vi "Manual User Input.vi"() -> (2 "XML":path, 3 "ZIP":path, 4 "Cancelled?":bool=TRUE)   [LabVIEW 2020]
doc: "<p>Select <strong>Tools<span class=\"U+187\">>></span>Synchronize with ni.com Icon Library</strong> from the <a href=\"nihelplauncher://docs/csh?context=lvcore_lvdialog_icon_editor\">Icon Editor</a> dialog box to display the <a href=\"nihelplauncher://docs/csh?context=lvcore_lvdialog_synch_icon_library_db\">Synchronize with Icon Library</a> dialog box. If LabVIEW cannot reach the National Instruments Web server, LabVIEW displays this dialog box.</p>\n\n<p>Use this dialog box to synchronize the <span class=\"Monospace\">LabVIEW Data\\Glyphs</span> directory <a href=\"nihelplauncher://docs/csh?context=lvcore_lvhowto_synchronizing_icon_library\">manually</a> with the most recent glyphs in the <a href=\"https://www.ni.com/r/expnr7\">Icon Library</a> at <span class=\"Monospace\">ni.com</span>.</p>\n\n<p>This dialog box includes the following components:</p>"
panel:
  in  "Loc string":string="LabVIEW cannot reach the National Instruments Web server. You must synchronize with the Icon Library manually.\nClick the Help button for more information about resolving this error."
  in  "Help":bool
  in  "Icon library XML file":path
  in  "Icon library ZIP file":path
  out "Instructions":string
  in  "Cancel":bool
  in  "OK":bool
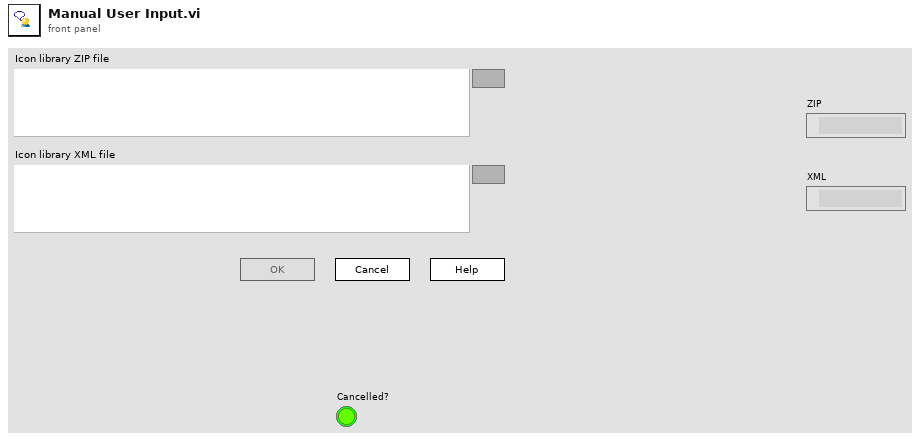
[diagram p1: front panel]
types:
  T1 = enum8{"Enabled", "Disabled", "Disabled and Grayed Out"}
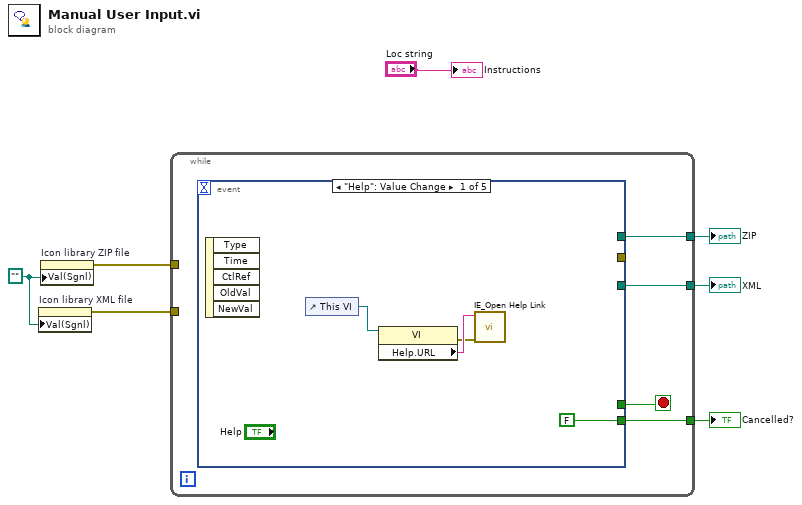
[diagram p0: block diagram]
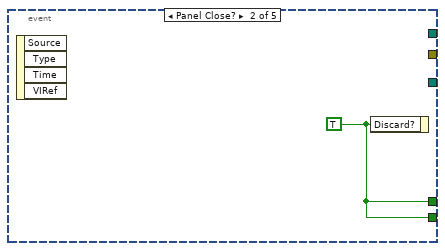
[diagram p2: hidden frame]
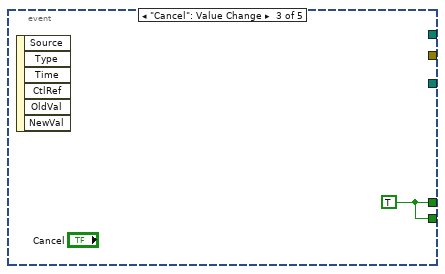
[diagram p3: hidden frame]
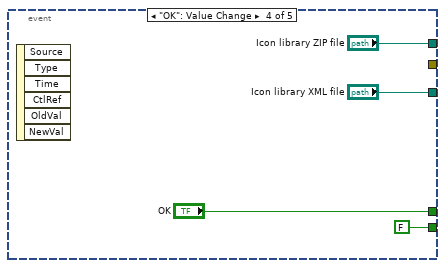
[diagram p4: hidden frame]
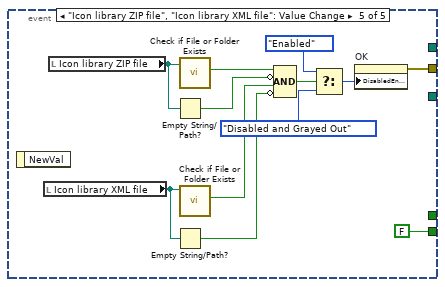
[diagram p5: hidden frame]
diagram:
  w5 = path ""
  n1 = property on="Icon library XML file" class="Path"("Val(Sgnl)"=w5) -> (error out=w2:errorcluster)  [unwired: 2 in, 1 out]
  n2 = property on="Icon library ZIP file" class="Path"("Val(Sgnl)"=w5) -> (error out=w3:errorcluster)  [unwired: 2 in, 1 out]
  n3 = while {
    tunnel: [w8] -> w7
    tunnel: [w11] -> w4
    tunnel: [w10] -> w6
    tunnel: w3 -> [_]
    tunnel: w2 -> [_]
    stop <- w9 stop-if-true
    n4 = event shown="[0] \"Help\": Value Change" {
      selector: _ -> [_ _ _ _ _]
      dyn-events: _ -> [_ _ _ _ _]
      timeout: _ -> [_ _ _ _ _]
      tunnel: [_ w16 w17 "OK" _] -> w9
      tunnel: [_ _ _ "Icon library ZIP file" _] -> w11
      tunnel: [_ _ _ "Icon library XML file" _] -> w10
      tunnel: [_ _ _ _ w23] -> _
      tunnel: [FALSE ("Discard?") w16 w17 FALSE ("Discard?") FALSE ("Discard?")] -> w8
      event "Help": Value Change {
        n5 = event-data() -> ()  [unwired: 1 in, 5 out]
        n6 = control-ref of="This VI"() -> (w14:refnum<vi>)
        n7 = property class="VI"(reference=w14) -> (error out=w12:errorcluster, "Help.URL"=w13:string)  [unwired: 1 in, 1 out]
        n8 = call "IE_Open Help Link.vi"("error in (no error)"=w12, "Help.URL"=w13) -> ()  [unwired: 9 in, 1 out]
      }
      event Panel Close? {
        w16 = TRUE ("Discard?")
        n9 = event-data() -> ()  [unwired: 1 in, 4 out]
        n10 = event-data("Discard?"=w16) -> ()  [unwired: 1 in, 1 out]
      }
      event "Cancel": Value Change {
        w17 = TRUE ("Discard?")
        n11 = event-data() -> ()  [unwired: 1 in, 6 out]
      }
      event "OK": Value Change {
        n12 = event-data() -> ()  [unwired: 1 in, 6 out]
      }
      event "Icon library ZIP file", "Icon library XML file": Value Change {
        n13 = event-data() -> ()  [unwired: 1 in, 1 out]
        n14 = local read "Icon library XML file"() -> (w32:path)
        n15 = local read "Icon library ZIP file"() -> (w33:path)
        n16 = Empty String/Path?(string/path=w33) -> (empty?=w30:bool)
        n17 = Empty String/Path?(string/path=w32) -> (empty?=w28:bool)
        n18 = call <vilib>:"Check if File or Folder Exists.vi"("path"=w33) -> ("file or folder exists?"=w31:bool)  [unwired: 8 in, 2 out]
        n19 = call <vilib>:"Check if File or Folder Exists.vi"("path"=w32) -> ("file or folder exists?"=w29:bool)  [unwired: 8 in, 2 out]
        n20 = Compound Arithmetic op=AND(w31, invert w30, w29, invert w28) -> (w27:bool)
        n21 = Select(t=T1."Enabled" ("Disabled"), s=w27, f=T1."Disabled and Grayed Out" ("Disabled")) -> (s? t:f=w26:T1)
        n22 = property on="OK" class="Bool"("DisabledEnum"=w26) -> (error out=w23:errorcluster)  [unwired: 2 in, 1 out]
      }
    }
  }
  "Cancelled?" <- w7
  "ZIP" <- w4
  "XML" <- w6
  "Instructions" <- "Loc string"
